vi "GetFrameworkConfigPath.vi"(8 "error in (no error)":errorcluster, 11 "SMO.UI.MAUI in":refnum<class "SMO.UI.MAUI.lvclass">) -> (0 "error out":errorcluster, 2 "Path":path, 3 "SMO.UI.MAUI out":refnum<class "SMO.UI.MAUI.lvclass">)   [LabVIEW 2019, in "SMO.UI.MAUI.lvclass"]
doc: "Provides a path to the framework's configuration file, which is located at %PublicApplicationData%\\maui\\maui_framework\\resource\\default.ini. If the folders for the file location do not exist, it will create them. Note: It will not create the file if it is not found."
uses:
  SMO.UI.MAUI.lvclass
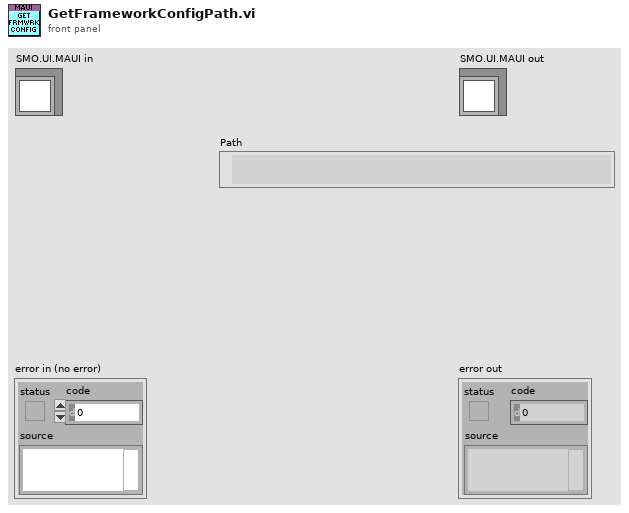
[diagram p1: front panel]
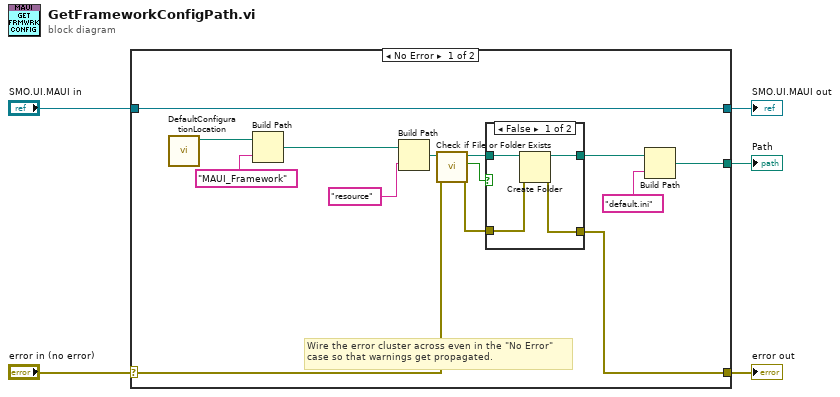
[diagram p0: block diagram]
diagram:
  n1 = case shown="No Error" "error in (no error)" {
    selector: "error in (no error)" -> [w8 w27]
    tunnel: [w6 w27] -> w4
    tunnel: [w19 w26] -> w2
    tunnel: "SMO.UI.MAUI in" -> [w19 w26]
    tunnel: [w13 _] -> w1
    frame No Error {
      # "Wire the error cluster across even in the \"No Error\"\ncase so that warnings get propagated."
      n2 = call "DefaultConfigurationLocation.vi"() -> ("DefaultConfigLocation"=w18:path)  [unwired: 11 in]
      n3 = Build Path(base path=w18, name or relative path="MAUI_Framework") -> (appended path=w16:path)
      n4 = Build Path(base path=w16, name or relative path="resource") -> (appended path=w12:path)
      n5 = call <vilib>:"Check if File or Folder Exists.vi"("error in (no error)"=w8, "path"=w12) -> ("error out"=w7:errorcluster, "file or folder exists?"=w9:bool, "dup path"=w11:path)  [unwired: 7 in]
      n6 = case shown="False" w9 {
        tunnel: w11 -> [w22 w24]
        tunnel: [w23 w24] -> w10
        tunnel: w7 -> [w21 w25]
        tunnel: [w20 w25] -> w6
        frame False {
          n7 = Create Folder(path (use dialog)=w22, error in=w21) -> (created path=w23:path, error out=w20:errorcluster)  [unwired: 1 in, 1 out]
        }
        frame True {
        }
      }
      n8 = Build Path(base path=w10, name or relative path="default.ini") -> (appended path=w13:path)
    }
    frame Error {
    }
  }
  "error out" <- w4
  "SMO.UI.MAUI out" <- w2
  "Path" <- w1
